vi "Read VAR.vi"(5 "Flow Meter DevID":i32=1, 7 "Timeout (ms)":u32, 8 "error in":errorcluster, 10 "Variable to Read":T1, 11 "VISA resource name":refnum<visa-resource-name>) -> (0 "error out":errorcluster, 1 "Read Buffer":string, 3 "VISA resource name out":refnum<visa-resource-name>)   [LabVIEW 2012, in "FEM-03.lvlib"]
uses:
  FEM-03.lvlib
  Private/Controls/Variable List.ctl
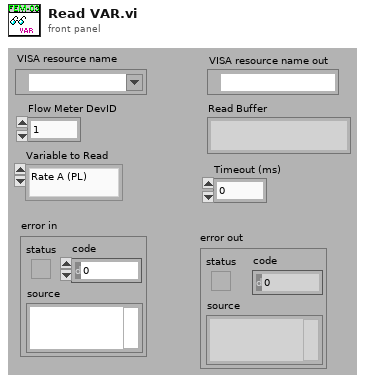
[diagram p1: front panel]
types:
  T1 = typedef "FEM-03.lvlib/Variable List.ctl" = enum16{"Rate A (PL)", "Rate A (GT)", "Job Total A", "Grand Total A", "A-KFR for Rate", "A-KFR decimal point location", "A-KFT for Total", "A-KFT decimal point location ", "A-Rate Engineering Units", "A-Total Engineering units", "A-Flow Direction", "Rate B (PL)", "Rate B (GT)", "Job Total B", "Grand Total B", "B-KFR for Rate", "B-KFR deciminal point location", "B-Rate Engineering units", "B-KFT for Total", "B-KFT decimal point location", "B-Total Engineering units", "Limit 1 Mode", "Limit1", "Margin 1 for rate limit", "Limit 2 Mode", "Limit2", "Margin 2 for rate limit", "Milli-amps Offset", "Milli-amps Out", "Analog Out Mode", "Serial Speed", "Unit Number", "Serial RESET TOTAL", "Update EEPROM", "Relay Override", "FORCE mA Output"}
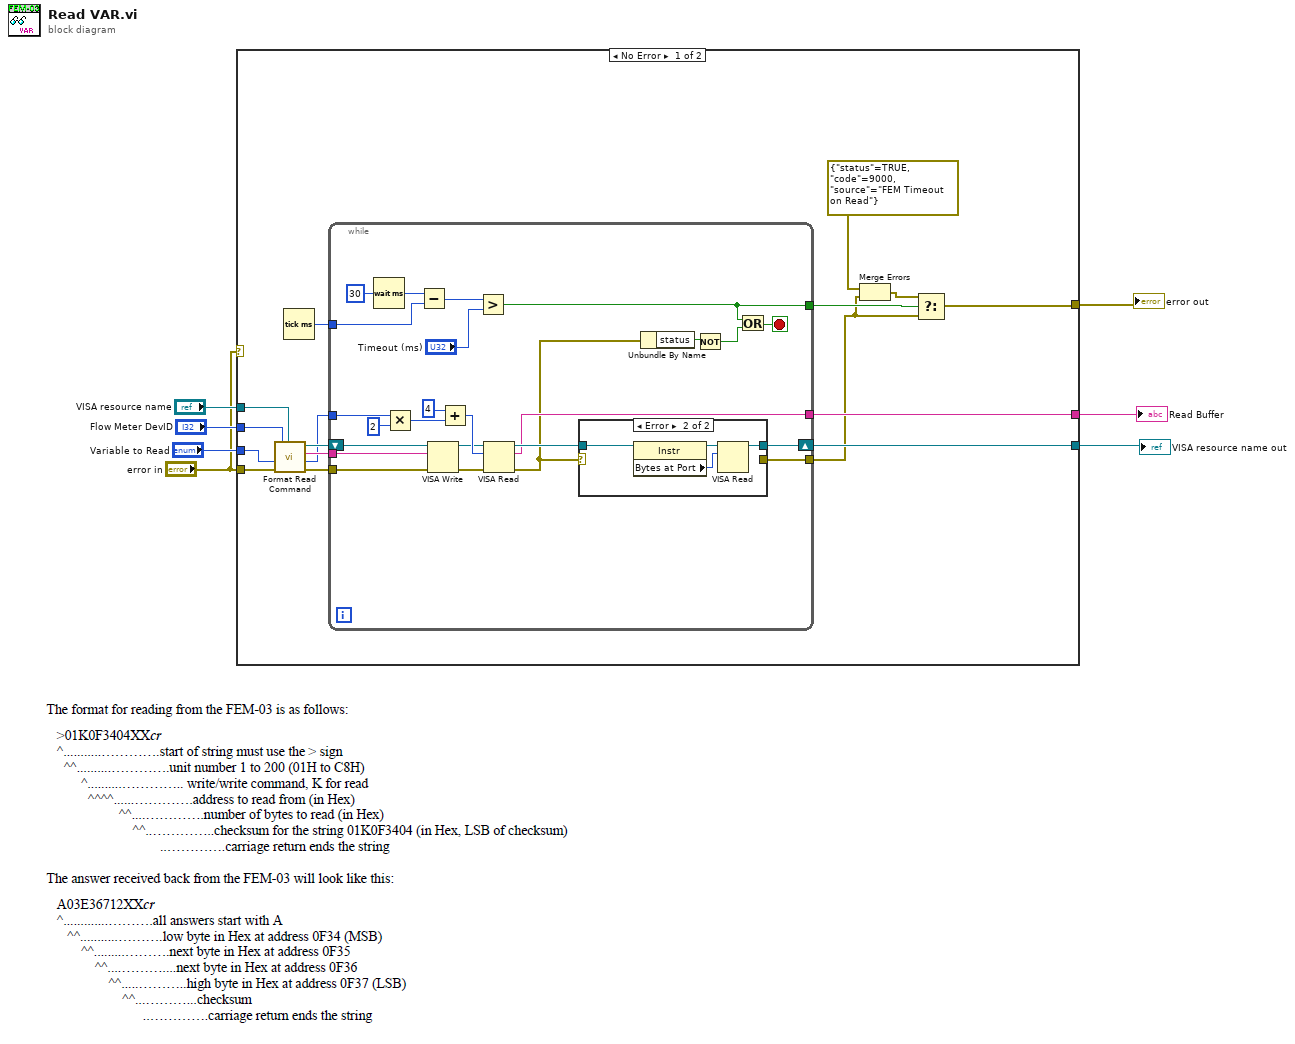
[diagram p0: block diagram]
diagram:
  n1 = case shown="No Error" "error in" {
    tunnel: "Flow Meter DevID" -> [w23 _]
    tunnel: "VISA resource name" -> [w19 w54]
    tunnel: "error in" -> [w18 w55]
    tunnel: [w16 _] -> w5
    tunnel: [w15 w54] -> w4
    tunnel: "Variable to Read" -> [w13 _]
    tunnel: [w11 w55] -> w2
    frame No Error {
      n2 = call "Format Read Command.vi"("error in"=w18, "Variable to Read"=w13, "Flow Meter DevID"=w23, "VISA resource name"=w19) -> ("error out"=w22:errorcluster, "Length Bytes (Dec)"=w17:i32, "Command String with Checksum"=w20:string, "VISA resource name out"=w21:refnum<visa-resource-name>)
      n3 = Tick Count (ms)() -> (millisecond timer value=w14:u32)
      n4 = while {
        tunnel: w22 -> [w47]
        tunnel: w20 -> [w45]
        tunnel: w17 -> [w44]
        shift-right: [w36] -> w15
        shift-left: w21 -> [w46]
        tunnel: [w35] -> w9
        tunnel: [w34] -> w16
        tunnel: w14 -> [w32]
        tunnel: [w26] -> w12
        stop <- w27 stop-if-true
        n5 = Wait (ms)(milliseconds to wait=u32 30) -> (millisecond timer value=w33:u32)
        n6 = Multiply(x=w44, y=2) -> (x*y=w42:i32)
        n7 = Subtract(x=w33, y=w32) -> (x-y=w30:u32)
        n8 = VISA Write(VISA resource name=w46, write buffer=w45, error in (no error)=w47) -> (VISA resource name out=w39:refnum<visa-resource-name>, error out=w38:errorcluster)  [unwired: 1 out]
        n9 = Add(x=4, y=w42) -> (x+y=w40:i32)
        n10 = Greater?(x=w30, y="Timeout (ms)") -> (0:w26:bool)
        n11 = VISA Read(VISA resource name=w39, byte count=w40, error in (no error)=w38) -> (VISA resource name out=w37:refnum<visa-resource-name>, read buffer=w34:string, error out=w25:errorcluster)  [unwired: 1 out]
        n12 = case shown="Error" w25 {
          selector: w25 -> [w49 _]
          tunnel: w37 -> [w48 w53]
          tunnel: [w48 w50] -> w36
          tunnel: [w49 _] -> w35
          frame No Error {
          }
          frame Error {
            n13 = property class="Instr"(reference=w53) -> (reference out=w52:refnum<visa-resource-name>, "Bytes at Port"=w51:u32)  [unwired: 1 in, 1 out]
            n14 = VISA Read(VISA resource name=w52, byte count=w51) -> (VISA resource name out=w50:refnum<visa-resource-name>)  [unwired: 1 in, 3 out]
          }
        }
        n15 = Unbundle By Name(w25) -> ("status"=w29:bool)
        n16 = Not(x=w29) -> (.not. x?=w28:bool)
        n17 = Or(x=w26, y=w28) -> (x .or. y?=w27:bool)
      }
      n18 = Merge Errors(errorcluster {"status"=TRUE, "code"=9000, "source"="FEM Timeout on Read"} ("error out"), w9) -> (w8:errorcluster)
      n19 = Select(t=w8, s=w12, f=w9) -> (s? t:f=w11:errorcluster)
    }
    frame Error {
    }
  }
  "Read Buffer" <- w5
  "VISA resource name out" <- w4
  "error out" <- w2
